vi "Global Counter count.vi"() -> ()   [LabVIEW 2020]
panel:
  in  "Global Counter count":dbl
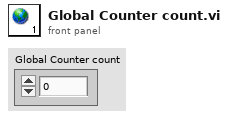
[diagram p1: front panel]
diagram:
